vi "Stream to TDMS Files (Optimized Performance).vi"() -> ()   [LabVIEW 2023]
doc: "The Stream to TDMS Files (Optimized Performance) example shows how to save images to a TDMS file when using a ring acquisition. The TDMS API has been optimized to take advantage of asynchronous writes, parallel background workers, disk reservation, and disabling buffering to improve write perfromance. Read the comments on the block diagram of this VI to learn more about these optimization options."
uses:
  <vilib>/vision/driver/IMAQdx.llb/IMAQdx Acquisition Mode.ctl
  SubVIs/TDMS Write Settings.ctl
  <vilib>/vision/Image Controls.llb/IMAQ Image.ctl
  <vilib>/vision/driver/IMAQdx.llb/IMAQdx Buffer Number Mode.ctl
  <vilib>/Utility/High Resolution Relative Seconds.vi
  SubVIs/TDMS File Initialization (Write).vi
  <vilib>/vision/EDVR.llb/IMAQ ImageToEDVR.vi
  <vilib>/vision/EDVR.llb/IMAQ ImageToEDVR 1D U8.vi
  <vilib>/vision/EDVR.llb/IMAQ ImageToEDVR 1D I16.vi
  <vilib>/vision/EDVR.llb/IMAQ ImageToEDVR 1D U32.vi
  <vilib>/vision/EDVR.llb/IMAQ ImageToEDVR 1D U16.vi
  <vilib>/vision/driver/NI_Vision_Acquisition_Software.lvlib
  <resource>/objmgr/imaqdx.rc
panel:
  out "Optimizations":T1
  in  "Skip Count":u32
  out "Images Saved Per Second":dbl
  out "Images Acquired Per Second":dbl
  in  "Images per TDMS":i64=10000
  out "Write Speed":dbl(graph) caption="Image File Write Speed"
  out "Destination Folder":path
  out "Images Behind":u32
  in  "Number of Images":i32=30
  in  "Camera Name":refnum<k21> caption="IMAQdx Session"
  in  "Stop":bool
  # "Overview: Demonstrates how to stream images to TDMS files when using a ring acquisition.\nRequirements: Vision Acquisition Software\nInstructions:\n1. Select the Camera Name\n2. Run the VI\n3. Increase the Skip Count if Images Behind is greater than 0."
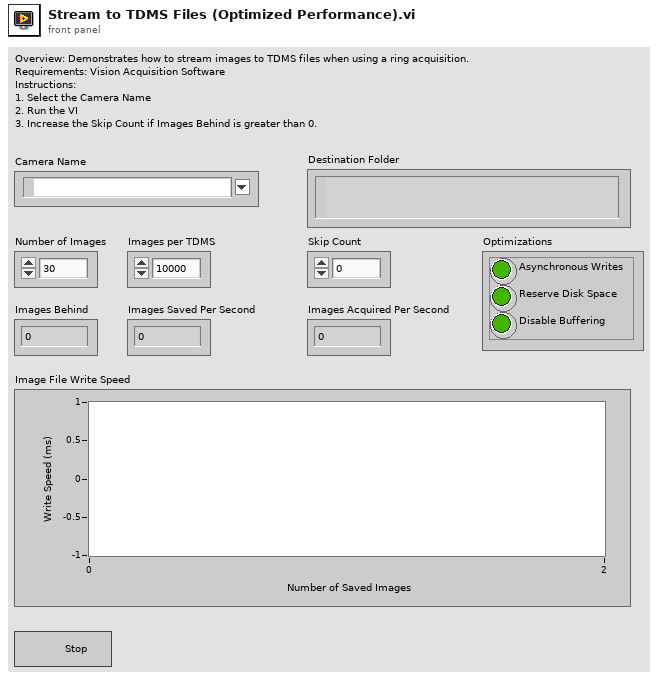
[diagram p1: front panel]
types:
  T1 = cluster{"Asynchronous Writes":bool, "Reserve Disk Space":bool, "Disable Buffering":bool}
  T2 = typedef "TDMS Write Settings.ctl" = cluster{"Asynchronous":bool, "Disable Buffering if Supported":bool, "Reserved Images":i64, "Fail if Reservation Fails":bool}
  T3 = typedef "NI_Vision_Acquisition_Software.lvlib/IMAQdx Acquisition Mode.ctl" = enum32{"One Shot", "Continuous"}
  T4 = typedef "IMAQdx.ctl" = refnum<k21>
  T5 = typedef "IMAQ Image.ctl" = refnum<image>
  T6 = typedef "Image Type" = u32
  T7 = cluster{"Image Type":T6, "Async File Format":bool}
  T8 = cluster{"Asynchronous Write":bool, "Reserve Disk Space":bool, "Disable Buffering":bool}
  T9 = typedef "NI_Vision_Acquisition_Software.lvlib/IMAQdx Buffer Number Mode.ctl" = enum32{"Next", "Last", "Buffer Number", "Every", "Last New"}
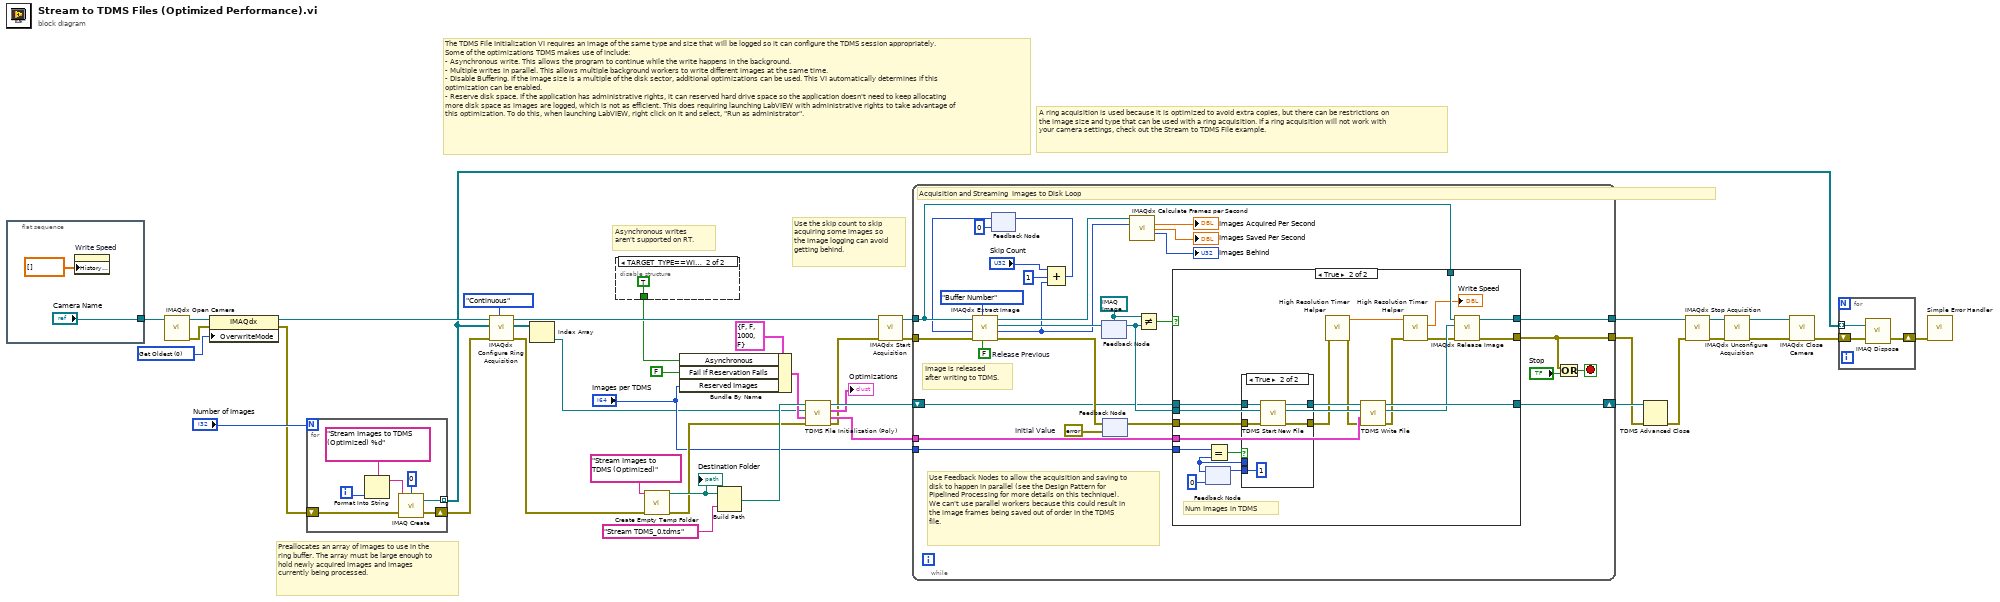
[diagram p0: block diagram]
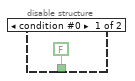
[diagram p2: hidden frame]
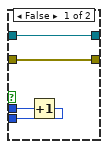
[diagram p4: hidden frame]
diagram:
  w11 = u32 0 items=["Get Oldest"=0, "Fail"=2, "Get Newest"=3] ("OverwriteMode")
  # "The TDMS File Initialization VI requires an image of the same type and size that will be logged so it can configure the TDMS session appropriately. Some of the optimizations TDMS makes use of include:\n- Asynchronous write. This allows the program to continue while the write happens in the background.\n- Multiple writes in parallel. This allows multiple background workers to write different images at the same time.\n- Disable Buffering. If the image size is a multiple of the disk sector, additional optimizations can be used. This VI automatically determines if this optimization can be enabled.\n- Reserve disk space. If the application has administrative rights, it can reserved hard drive space so the application doesn't need to keep allocating more disk space as images are logged, which is not as efficient. This does requiring launching LabVIEW with administrative rights to take advantage of this optimization. To do this, when launching LabVIEW, right click on it and select, \"Run as administrator\"."
  # "Asynchronous writes aren't supported on RT."
  # "Use the skip count to skip acquiring some images so the image logging can avoid getting behind."
  # "A ring acquisition is used because it is optimized to avoid extra copies, but there can be restrictions on the image size and type that can be used with a ring acquisition. If a ring acquisition will not work with your camera settings, check out the Stream to TDMS File example."
  # "Preallocates an array of images to use in the ring buffer. The array must be large enough to hold newly acquired images and images currently being processed."
  n1 = flat-sequence {
    tunnel: ["Camera Name"] -> w40
    frame #0 {
      n2 = property on="Write Speed" class="WFChart (strict)"("History Data"=dbl[] []) -> ()  [unwired: 2 in, 2 out]
    }
  }
  n3 = call <vilib>:"IMAQdx Open Camera.vi"("Session In"=w40) -> ("error out"=w35:errorcluster, "Session Out"=w36:T4)  [unwired: 2 in, 7 out]
  n4 = property class="IMAQdx"(reference=w36, error in=w35, "OverwriteMode"=w11) -> (reference out=w33:T4, error out=w7:errorcluster)
  n5 = for {
    N: "Number of Images" -> [_]
    tunnel: [w48] -> w6 mode=indexing
    shift-right: [w47] -> w5
    shift-left: w7 -> [w49]
    i -> [w46]
    n6 = Format Into String(format string="Stream Images to TDMS (Optimized) %d" ("Image Name"), w46) -> (resulting string=w45:string)  [unwired: 2 in, 1 out]
    n7 = call "IMAQ Create"("Border Size"=0, "Image Name"=w45, "error in (no error)"=w49) -> ("New Image"=w48:T5, "error out"=w47:errorcluster)  [unwired: 1 in, 1 out]
  }
  n8 = call <vilib>:"IMAQdx Configure Ring Acquisition.vi"("Mode"=IMAQdx_Acquisition_Mode."Continuous" ("Continuous?"), "error in"=w5, "Images"=w6, "Session In"=w33) -> ("error out"=w4:errorcluster, "Images Out"=w3:T5[], "Session Out"=w30:T4)  [unwired: 5 in]
  n9 = Index Array(array=w3) -> (element=w2:T5)  [unwired: 1 in]
  n10 = disable-structure shown="TARGET_TYPE==Windows" {
    disable-tunnel: [FALSE ("Asynchronous") TRUE ("Asynchronous")] -> w13
    frame condition #0 {
    }
    frame condition #1 (active) {
    }
  }
  n11 = call "Create Empty Temp Folder.vi"("error in (no error)"=w4, "Folder Name"="Stream Images to TDMS (Optimized)") -> ("error out"=w20:errorcluster, "Empty Temp Folder"=w24:path)  [unwired: 8 in]
  "Destination Folder" <- w24
  n12 = Bundle By Name(cluster=T2 {"Asynchronous"=FALSE, "Disable Buffering if Supported"=FALSE, "Reserved Images"=1000, "Fail if Reservation Fails"=FALSE} ("Write Settings"), "Asynchronous"=w13, "Fail if Reservation Fails"=FALSE, "Reserved Images"="Images per TDMS") -> (w12:T2)
  n13 = Build Path(base path=w24, name or relative path="Stream TDMS_0.tdms") -> (appended path=w21:path)
  n14 = call-poly "TDMS File Initialization (Poly).vi"("error in (no error)"=w20, "Write Settings"=w12, "Image In"=w2, "File Path"=w21) -> ("error out"=w1:errorcluster, "Write Settings Out"=w18:T7, "Optimizations Configured"=→"Optimizations":T8, "TDMS Refnum Out"=w22:refnum<k34>)  [unwired: 4 in]
  n15 = call <vilib>:"IMAQdx Start Acquisition.vi"("error in"=w1, "Session In"=w30) -> ("error out"=w26:errorcluster, "Session Out"=w27:T4)  [unwired: 8 out]
  n16 = while {
    tunnel: w26 -> [w80]
    tunnel: w27 -> [w76]
    tunnel: [w77] -> w28
    tunnel: [w65] -> w16
    shift-right: [w78] -> w17
    shift-left: w22 -> [w62]
    tunnel: "Images per TDMS" -> [w61]
    tunnel: w18 -> [w64]
    stop <- w67 stop-if-true
    w52 = errorcluster {"status"=FALSE, "code"=0, "source"=""}  # Initial Value
    w74 = FALSE  # Release Previous
    w70 = T5 refnum ("Image Out")
    # "Use Feedback Nodes to allow the acquisition and saving to disk to happen in parallel (see the Design Pattern for Pipelined Processing for more details on this technique). We can't use parallel workers because this could result in the image frames being saved out of order in the TDMS file."
    # "Image is released after writing to TDMS."
    # "Acquisition and Streaming  Images to Disk Loop"
    n17 = feedback #1(u32 0) -> (w54:u32)
    n18 = call <vilib>:"IMAQdx Extract Image.vi"("Release Previous (true)"=w74, "Buffer Number Mode (Next)"=IMAQdx_Buffer_Number_Mode."Buffer Number" ("Buffer Number Mode"), "error in"=w80, "Buffer Number In"=w54, "Session In"=w76) -> ("error out"=w63:errorcluster, "Buffer Number Out"=w56:u32, "Image Out"=w72:T5, "Session Out"=w73:T4)  [unwired: 3 in]
    n19 = Compound Arithmetic op=ADD("Skip Count", u32 1 ("value"), w56) -> (w57:u32)
    n20 = feedback-in #1(w57) -> ()
    n21 = feedback-in #2(w72) -> ()
    n22 = feedback #2(w70) -> (w68:T5)
    n23 = feedback-in #3(w63) -> ()
    n24 = feedback #3(w52) -> (w71:errorcluster)
    n25 = call <vilib>:"IMAQdx Calculate Frames per Second.vi"("Session In"=w73, "Buffer Number"=w56) -> ("Acquired Frames per Second"=→"Images Acquired Per Second":dbl, "Processed Frames per Second"=→"Images Saved Per Second":dbl, "Images Behind"=→"Images Behind":i32)  [unwired: 7 in, 4 out]
    n26 = Not Equal?(x=w70, y=w68) -> (x != y?=w69:bool)
    n27 = case shown="True" w69 {
      tunnel: w62 -> [w81 w96]
      tunnel: w68 -> [_ w98]
      tunnel: w71 -> [w82 w94]
      tunnel: [w81 w100] -> w78
      tunnel: [w83 w103] -> w77
      tunnel: w76 -> [w83 w102]
      tunnel: [w82 w101] -> w65
      tunnel: w64 -> [_ w99]
      tunnel: w61 -> [_ w92]
      frame False {
        # "First iteration doesn't have valid image for this pipelined stage."
      }
      frame True {
        # "Num Images in TDMS"
        n28 = feedback #4(i64 0) -> (w91:i64)
        n29 = Equal?(x=w92, y=w91) -> (x = y?=w93:bool)
        n30 = case shown="True" w93 {
          tunnel: [w107 i64 1] -> w90
          tunnel: w96 -> [w106 w111]
          tunnel: [w106 w110] -> w95
          tunnel: w94 -> [w105 w108]
          tunnel: [w105 w109] -> w89
          tunnel: w91 -> [w104 _]
          frame False {
            n31 = Increment(x=w104) -> (x+1=w107:i64)
          }
          frame True {
            n32 = call "TDMS Start New File.vi"("error in"=w108, "Previous TDMS Refnum In"=w111) -> ("error out"=w109:errorcluster, "New TDMS Refnum Out"=w110:refnum<k34>)  [unwired: 8 in]
          }
        }
        n33 = feedback-in #4(w90) -> ()
        n34 = call "High Resolution Timer Helper.vi"("error in (no error)"=w89) -> ("error out"=w88:errorcluster, "Current Time"=w86:dbl)  [unwired: 8 in, 1 out]
        n35 = call "TDMS Write File.vi"("error in"=w88, "Write Settings"=w99, "Image"=w98, "TDMS Ref In"=w95) -> ("error out"=w87:errorcluster, "TDMS Ref Out"=w100:refnum<k34>)  [unwired: 6 in]
        n36 = call "High Resolution Timer Helper.vi"("error in (no error)"=w87, "Previous Time"=w86) -> ("error out"=w85:errorcluster, "Time Difference (ms)"=→"Write Speed":dbl)  [unwired: 7 in, 1 out]
        n37 = call <vilib>:"IMAQdx Release Image.vi"("error in"=w85, "Image"=w98, "Session In"=w102) -> ("error out"=w101:errorcluster, "Session Out"=w103:T4)  [unwired: 7 in]
      }
    }
    n38 = Or(x=w65, y="Stop") -> (x .or. y?=w67:bool)
  }
  n39 = TDMS Advanced Close(8:w16, 11:w17) -> (0:w15:errorcluster)  [unwired: 2 in, 1 out]
  n40 = call <vilib>:"IMAQdx Stop Acquisition.vi"("error in"=w15, "Session In"=w28) -> ("error out"=w31:errorcluster, "Session Out"=w32:T4)  [unwired: 8 out]
  n41 = call <vilib>:"IMAQdx Unconfigure Acquisition.vi"("error in"=w31, "Session In"=w32) -> ("error out"=w39:errorcluster, "Session Out"=w38:T4)  [unwired: 8 out]
  n42 = call <vilib>:"IMAQdx Close Camera.vi"("error in"=w39, "Session In"=w38) -> ("error out"=w34:errorcluster)  [unwired: 9 out]
  n43 = for {
    shift-right: [w114] -> w8
    shift-left: w34 -> [w115]
    tunnel: w6 -> [w113] mode=indexing
    n44 = call "IMAQ Dispose"("Image"=w113, "error in (no error)"=w115) -> ("error out"=w114:errorcluster)  [unwired: 4 in]
  }
  n45 = call <vilib>:"Simple Error Handler.vi"("error in (no error)"=w8) -> ()  [unwired: 4 in, 5 out]
